vi "LRange.vi"(0 "reference in":refnum<class "RedisConnection.lvclass">, 1 "Key":string, 5 "Start":string, 9 "Stop":string, 11 "Error In":errorcluster) -> (4 "reference out":refnum<class "RedisConnection.lvclass">, 8 "Data":T1, 15 "Error Out":errorcluster)   [LabVIEW 2020, in "RedisConnection.lvclass"]
doc: "<b>LRANGE</b>\n\nReturns the specified elements of the list stored at key. The offsets start and stop are zero-based indexes, with 0 being the first element of the list (the head of the list), 1 being the next element and so on.\n\nThese offsets can also be negative numbers indicating offsets starting at the end of the list. For example, -1 is the last element of the list, -2 the penultimate, and so on."
uses:
  RedisConnection.lvclass
  RedisConnection.lvclass/RedisConnection.ctl
  ReplyDataTypeEnum.ctl
  RedisDataType.ctl
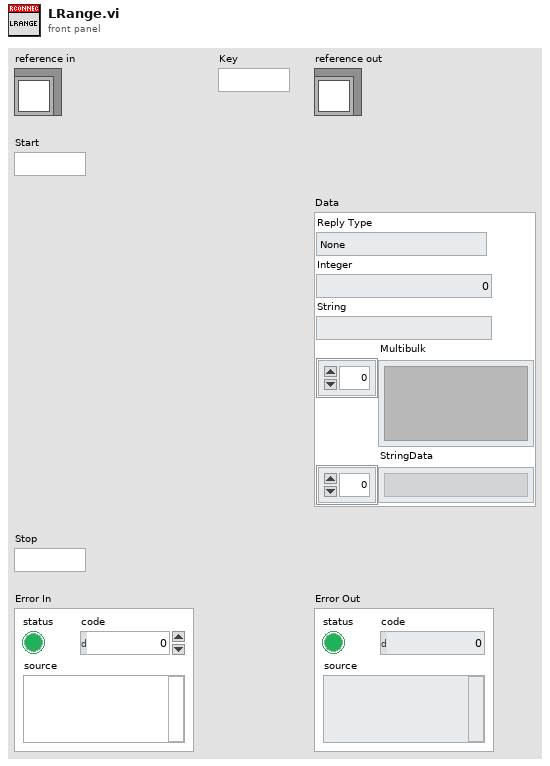
[diagram p1: front panel]
types:
  T1 = typedef "RedisConnection.lvclass/RedisDataType.ctl" = cluster{"Reply Type":T2, "Integer":i64, "String":string, "Multibulk":variant[], "StringData":string[]}
  T2 = typedef "RedisConnection.lvclass/ReplyDataTypeEnum.ctl" = enum16{"None", "Error", "Status", "Nil", "Integer", "String", "Multibulk"}
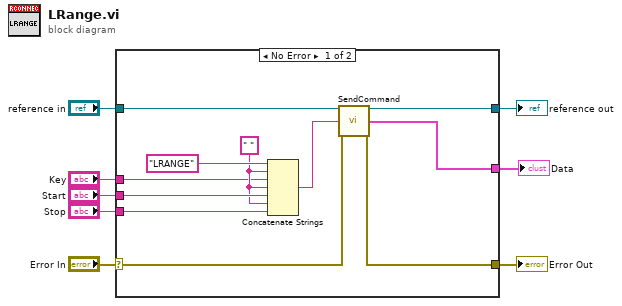
[diagram p0: block diagram]
diagram:
  n1 = case shown="No Error" "Error In" {
    selector: "Error In" -> [w17 w21]
    tunnel: [w16 w21] -> w7
    tunnel: [w19 w20] -> w5
    tunnel: "reference in" -> [w18 w20]
    tunnel: [w15 _] -> w4
    tunnel: "Start" -> [w13 _]
    tunnel: "Stop" -> [w11 _]
    tunnel: "Key" -> [w9 _]
    frame No Error {
      w10 = " "
      n2 = Concatenate Strings("LRANGE", w10, w9, w10, w13, w10, w11) -> (w12:string)
      n3 = call "SendCommand.vi"("reference in"=w18, "Command"=w12, "Error In"=w17) -> ("reference out"=w19:refnum<class "RedisConnection.lvclass">, "Data"=w15:T1, "Error Out"=w16:errorcluster)  [unwired: 10 in]
    }
    frame Error {
    }
  }
  "Error Out" <- w7
  "reference out" <- w5
  "Data" <- w4
